vi "FPGA_convert_pannel-channel-to-U16-v0.vi"(1 "pannel|channel":u16) -> (0 "Numérique":u16)   [LabVIEW 2010]
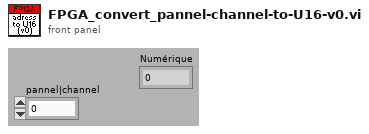
[diagram p1: front panel]
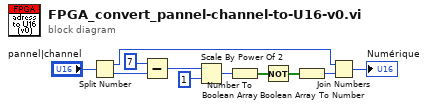
[diagram p0: block diagram]
diagram:
  n1 = Split Number(x="pannel|channel") -> (hi(x)=w3:u8, lo(x)=w4:u8)
  n2 = Subtract(x=u8 7, y=w4) -> (x-y=w6:u8)
  n3 = Scale By Power Of 2(n=w6, x=u8 1) -> (x*2^n=w8:u8)
  n4 = Number To Boolean Array(number=w8) -> (Boolean array=w9:bool[])
  n5 = Not(x=w9) -> (.not. x?=w10:bool[])
  n6 = Boolean Array To Number(Boolean array=w10) -> (number=w11:u8)
  n7 = Join Numbers(hi=w3, lo=w11) -> ((hi.lo)=→"Numérique":u16)
